vi "#74_MAV_MSG_VFR_HUD_DECODE.vi"(11 "mavlink_payload":u8[](array[numeric])) -> (3 "VFR_HUD":T1)   [LabVIEW 2023]
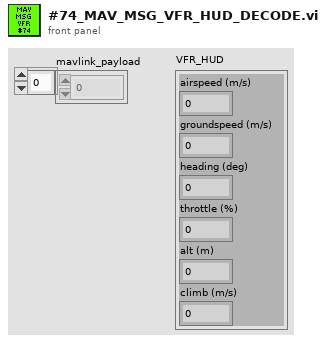
[diagram p1: front panel]
types:
  T1 = cluster{"airspeed (m/s)":sgl, "groundspeed (m/s)":sgl, "heading (deg) ":i16, "throttle (%) ":u16, "alt (m)":sgl, "climb (m/s)":sgl}
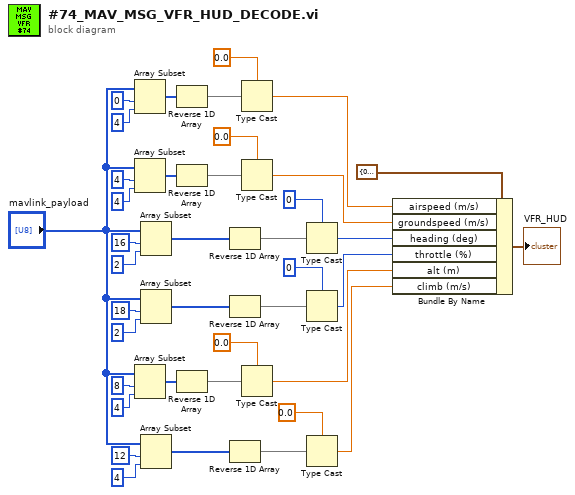
[diagram p0: block diagram]
diagram:
  n1 = Array Subset(array="mavlink_payload", index=0 ("Index"), length=4) -> (w38:u8[])
  n2 = Array Subset(array="mavlink_payload", index=4 ("Index"), length=4) -> (w31:u8[])
  n3 = Array Subset(array="mavlink_payload", index=8 ("Index"), length=4) -> (w12:u8[])
  n4 = Array Subset(array="mavlink_payload", index=16 ("Index"), length=2) -> (w26:u8[])
  n5 = Array Subset(array="mavlink_payload", index=18 ("Index"), length=2) -> (w21:u8[])
  n6 = Array Subset(array="mavlink_payload", index=12 ("Index"), length=4) -> (w6:u8[])
  n7 = Reverse 1D Array(array=w38) -> (reversed array=w37:u8[])
  n8 = Reverse 1D Array(array=w31) -> (reversed array=w30:u8[])
  n9 = Reverse 1D Array(array=w12) -> (reversed array=w11:u8[])
  n10 = Reverse 1D Array(array=w26) -> (reversed array=w25:u8[])
  n11 = Reverse 1D Array(array=w21) -> (reversed array=w20:u8[])
  n12 = Reverse 1D Array(array=w6) -> (reversed array=w5:u8[])
  n13 = Type Cast(type=sgl 0.0 ("Index"), x=w37) -> (*(type *) &x=w17:sgl)
  n14 = Type Cast(type=sgl 0.0 ("Index"), x=w30) -> (*(type *) &x=w16:sgl)
  n15 = Type Cast(type=sgl 0.0 ("Index"), x=w11) -> (*(type *) &x=w8:sgl)
  n16 = Type Cast(type=i16 0 ("Index"), x=w25) -> (*(type *) &x=w15:i16)
  n17 = Type Cast(type=u16 0 ("Index"), x=w20) -> (*(type *) &x=w14:u16)
  n18 = Type Cast(type=sgl 0.0 ("Index"), x=w5) -> (*(type *) &x=w1:sgl)
  n19 = Bundle By Name(cluster=T1 {"airspeed (m/s)"=0.0, "groundspeed (m/s)"=0.0, "heading (deg) "=0, "throttle (%) "=0, "alt (m)"=0.0, "climb (m/s)"=0.0} ("VFR_HUD"), "airspeed (m/s)"=w17, "groundspeed (m/s)"=w16, "heading (deg)"=w15, "throttle (%)"=w14, "alt (m)"=w8, "climb (m/s)"=w1) -> (→"VFR_HUD":T1)
